vi "QSPARK_fireLaser.vi"(11 "client handle":T1) -> (3 "client handle out":T1)   [LabVIEW 2024]
uses:
  <vilib>/httpClient/LabVIEWHTTPClient.lvlib
  <vilib>/httpClient/ClientHandle.ctl
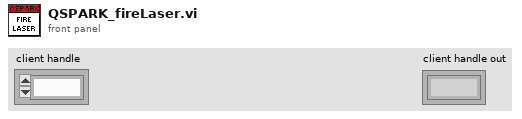
[diagram p1: front panel]
types:
  T1 = typedef "LabVIEWHTTPClient.lvlib/ClientHandle.ctl" = refnum<k1>
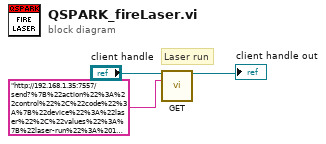
[diagram p0: block diagram]
diagram:
  # "Laser run"
  n1 = call <vilib>:"GET.vi"("client handle"="client handle", "url"="http://192.168.1.35:7557/send?%7B%22action%22%3A%22control%22%2C%22code%22%3A%7B%22device%22%3A%22laser%22%2C%22values%22%3A%7B%22laser-run%22%3A%201%7D%7D%7D") -> ("client handle out"=→"client handle out":T1)  [unwired: 10 in, 3 out]
